vi "KepcoDCPwr Configure List Count.vi"(0 "VISA Session":refnum<visa-resource-name>, 1 "# of Cycles":i32=1 min=0 max=255, 5 "Model In":string, 7 "channel name (\"\")":string="\"\"", 11 "error in (no error)":errorcluster {"code" format="%.0x"}) -> (4 "VISA Session Out":refnum<visa-resource-name>, 6 "Model Out":string, 8 "channel name out (\"\")":string="\"\"" caption="channel name Out (\"\")", 15 "error out":errorcluster {"code" format="%.0x"})   [LabVIEW 2013]
doc: "This VI Sets List count to value provided.\n\nNote:\n\n1) This VI does not change operational status of Power supply\n2. This Vi should be used before starting list.\n3.) clear list sets count to 1"
uses:
  <vilib>/regexp/Match Regular Expression.xnode
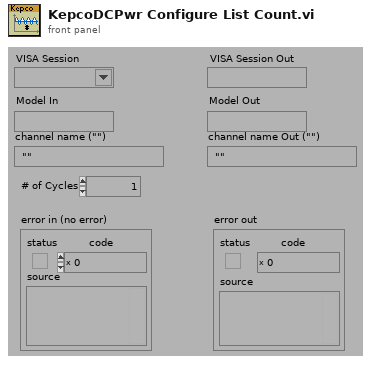
[diagram p1: front panel]
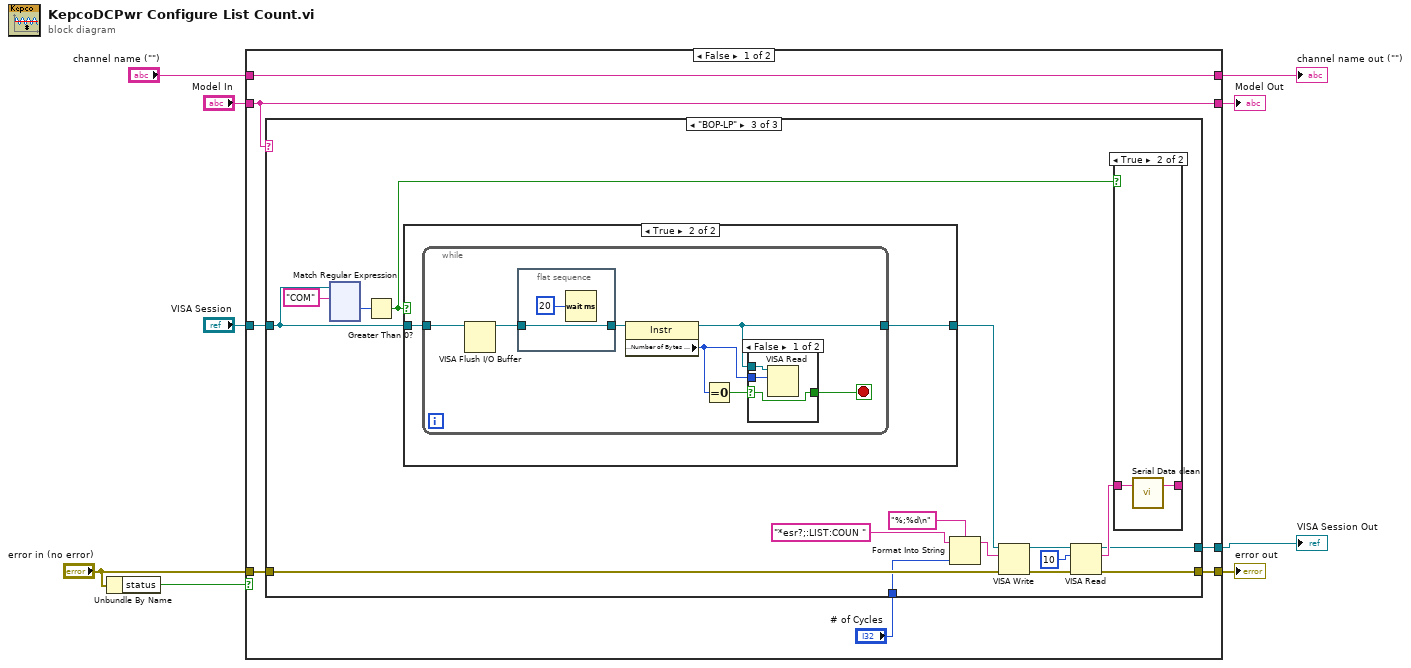
[diagram p0: block diagram]
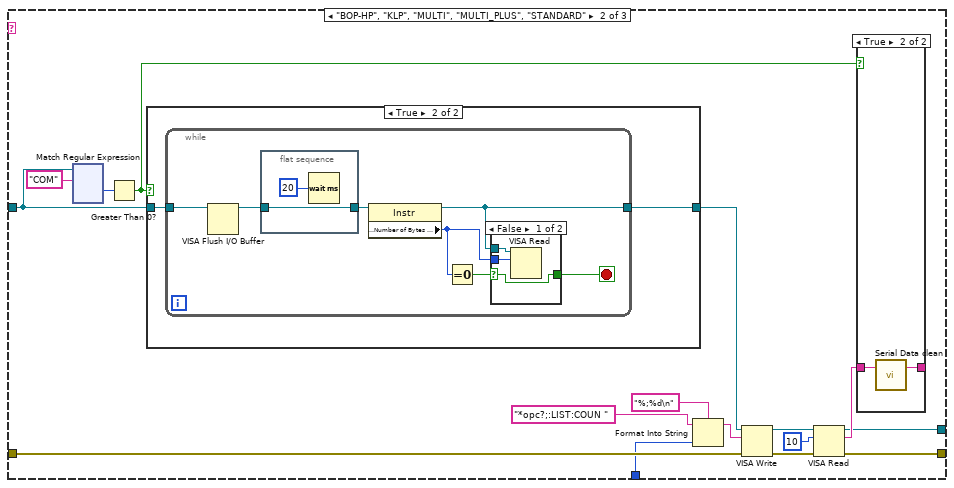
[diagram p3: hidden frame]
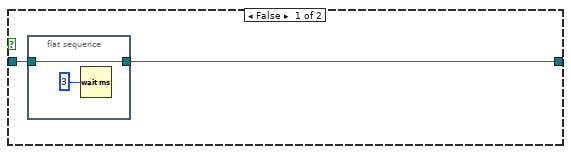
[diagram p5: hidden frame]
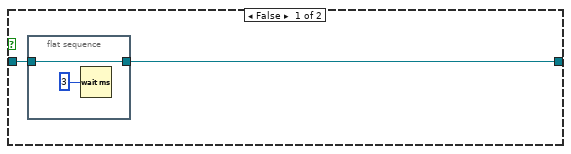
[diagram p8: hidden frame]
diagram:
  n1 = Unbundle By Name("error in (no error)") -> ("status"=w8:bool)
  n2 = case shown="False" w8 {
    tunnel: [w12 w320] -> w9
    tunnel: "error in (no error)" -> [w11 w320]
    tunnel: [w13 w319] -> w1
    tunnel: "VISA Session" -> [w14 w319]
    tunnel: [w15 w318] -> w2
    tunnel: "Model In" -> [w15 w318]
    tunnel: [w16 w317] -> w3
    tunnel: "channel name (\"\")" -> [w16 w317]
    frame False {
      n3 = case shown="\"BOP-LP\"" w15 {
        tunnel: w11 -> [w18 w27 w176]
        tunnel: [w18 w21 w170] -> w12
        tunnel: w14 -> [w17 w32 w181]
        tunnel: [w17 w22 w171] -> w13
        tunnel: "# of Cycles" -> [_ w19 w168]
        frame "", Default {
        }
        frame "BOP-HP", "KLP", "MULTI", "MULTI_PLUS", "STANDARD" {
          n4 = xnode "Match Regular Expression"("input string"=w32, "regular expression"="COM") -> ("offset past match"=w33:i32)  [unwired: 2 in, 6 out]
          n5 = Greater Than 0?(x=w33) -> (x > 0?=w31:bool)
          n6 = case shown="True" w31 {
            tunnel: [w39 w43] -> w28
            tunnel: w32 -> [w38 w42]
            frame False {
              n7 = flat-sequence {
                tunnel: w38 -> [w41]
                tunnel: [w41] -> w39
                frame #0 {
                  n8 = Wait (ms)(milliseconds to wait=u32 3 ("byte count (0)")) -> ()  [unwired: 1 out]
                }
              }
            }
            frame True {
              n9 = while {
                tunnel: w42 -> [w46]
                tunnel: [w48] -> w43
                stop <- w49 stop-if-true
                n10 = VISA Flush I/O Buffer(VISA resource name=w46) -> (VISA resource name out=w45:refnum<visa-resource-name>)  [unwired: 2 in, 1 out]
                n11 = flat-sequence {
                  tunnel: w45 -> [w51]
                  tunnel: [w51] -> w44
                  frame #0 {
                    n12 = Wait (ms)(milliseconds to wait=u32 20) -> ()  [unwired: 1 out]
                  }
                }
                n13 = property class="Instr"(reference=w44) -> (reference out=w48:refnum<visa-resource-name>, "Serial Settings:Number of Bytes at Serial Port"=w47:u32)  [unwired: 1 in, 1 out]
                n14 = Equal To 0?(x=w47) -> (x = 0?=w50:bool)
                n15 = case shown="False" w50 {
                  selector: w50 -> [w55 w56]
                  tunnel: [w55 w56] -> w49
                  tunnel: w48 -> [w54 _]
                  tunnel: w47 -> [w53 _]
                  frame False {
                    n16 = VISA Read(VISA resource name=w54, byte count=w53) -> ()  [unwired: 1 in, 4 out]
                  }
                  frame True {
                  }
                }
              }
            }
          }
          n17 = Format Into String(format string="%;%d\n", initial string="*opc?;:LIST:COUN ", w19) -> (resulting string=w29:string)  [unwired: 1 in, 1 out]
          n18 = VISA Write(VISA resource name=w28, write buffer=w29, error in (no error)=w27) -> (VISA resource name out=w26:refnum<visa-resource-name>, error out=w25:errorcluster)  [unwired: 1 out]
          n19 = VISA Read(VISA resource name=w26, byte count=u32 10, error in (no error)=w25) -> (VISA resource name out=w22:refnum<visa-resource-name>, read buffer=w23:string, error out=w21:errorcluster)  [unwired: 1 out]
          n20 = case shown="True" w31 {
            tunnel: w23 -> [w35 w36]
            tunnel: [w35 w37] -> _
            frame False {
            }
            frame True {
              n21 = call "Serial Data clean.vi"("string"=w36) -> ("Stripped of Xon Xoff"=w37:string)  [unwired: 2 in]
            }
          }
        }
        frame "BOP-LP" {
          n22 = xnode "Match Regular Expression"("input string"=w181, "regular expression"="COM") -> ("offset past match"=w182:i32)  [unwired: 2 in, 6 out]
          n23 = Greater Than 0?(x=w182) -> (x > 0?=w180:bool)
          n24 = case shown="True" w180 {
            tunnel: [w188 w192] -> w177
            tunnel: w181 -> [w187 w191]
            frame False {
              n25 = flat-sequence {
                tunnel: w187 -> [w190]
                tunnel: [w190] -> w188
                frame #0 {
                  n26 = Wait (ms)(milliseconds to wait=u32 3 ("byte count (0)")) -> ()  [unwired: 1 out]
                }
              }
            }
            frame True {
              n27 = while {
                tunnel: w191 -> [w195]
                tunnel: [w197] -> w192
                stop <- w198 stop-if-true
                n28 = VISA Flush I/O Buffer(VISA resource name=w195) -> (VISA resource name out=w194:refnum<visa-resource-name>)  [unwired: 2 in, 1 out]
                n29 = flat-sequence {
                  tunnel: w194 -> [w200]
                  tunnel: [w200] -> w193
                  frame #0 {
                    n30 = Wait (ms)(milliseconds to wait=u32 20) -> ()  [unwired: 1 out]
                  }
                }
                n31 = property class="Instr"(reference=w193) -> (reference out=w197:refnum<visa-resource-name>, "Serial Settings:Number of Bytes at Serial Port"=w196:u32)  [unwired: 1 in, 1 out]
                n32 = Equal To 0?(x=w196) -> (x = 0?=w199:bool)
                n33 = case shown="False" w199 {
                  selector: w199 -> [w204 w205]
                  tunnel: [w204 w205] -> w198
                  tunnel: w197 -> [w203 _]
                  tunnel: w196 -> [w202 _]
                  frame False {
                    n34 = VISA Read(VISA resource name=w203, byte count=w202) -> ()  [unwired: 1 in, 4 out]
                  }
                  frame True {
                  }
                }
              }
            }
          }
          n35 = Format Into String(format string="%;%d\n", initial string="*esr?;:LIST:COUN ", w168) -> (resulting string=w178:string)  [unwired: 1 in, 1 out]
          n36 = VISA Write(VISA resource name=w177, write buffer=w178, error in (no error)=w176) -> (VISA resource name out=w175:refnum<visa-resource-name>, error out=w174:errorcluster)  [unwired: 1 out]
          n37 = VISA Read(VISA resource name=w175, byte count=u32 10, error in (no error)=w174) -> (VISA resource name out=w171:refnum<visa-resource-name>, read buffer=w172:string, error out=w170:errorcluster)  [unwired: 1 out]
          n38 = case shown="True" w180 {
            tunnel: w172 -> [w184 w185]
            tunnel: [w184 w186] -> _
            frame False {
            }
            frame True {
              n39 = call "Serial Data clean.vi"("string"=w185) -> ("Stripped of Xon Xoff"=w186:string)  [unwired: 2 in]
            }
          }
        }
      }
    }
    frame True {
    }
  }
  "error out" <- w9
  "channel name out (\"\")" <- w3
  "Model Out" <- w2
  "VISA Session Out" <- w1
